vi "VisitLVType.vi"(8 "error in (no error)":errorcluster, 10 "LVType":refnum<class "LVType.lvclass">, 11 "NextGenXMLTypeGenerator in":refnum<class "NextGenXMLTypeGenerator.lvclass">) -> (0 "error out":errorcluster, 3 "NextGenXMLTypeGenerator out":refnum<class "NextGenXMLTypeGenerator.lvclass">)   [LabVIEW 2020, in "Web Service Description.lvlib" / "NextGenXMLTypeGenerator.lvclass"]
uses:
  <vilib>/AppBuilder/Engine/WebServiceDescription/NextGenXMLTypeGenerator/NextGenXMLTypeGenerator.lvclass
  <vilib>/AppBuilder/Engine/WebServiceDescription/LVDataTypes/LVType/LVType.lvclass
  <vilib>/AppBuilder/Engine/WebServiceDescription/XMLGen/ValuePair.ctl
  <vilib>/AppBuilder/Engine/WebServiceDescription/NextGenXMLTypeGenerator/NextGenXMLTypeGenerator.lvclass/NextGenXMLTypeGenerator.ctl
  <vilib>/AppBuilder/Engine/WebServiceDescription/XMLGen/XMLGen.lvlib
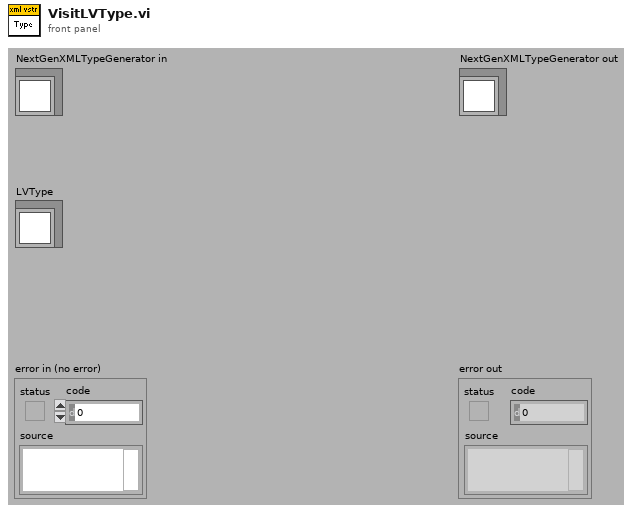
[diagram p1: front panel]
types:
  T1 = typedef "XMLGen.lvlib/ValuePair.ctl" = cluster{"Name":string, "Value":string}
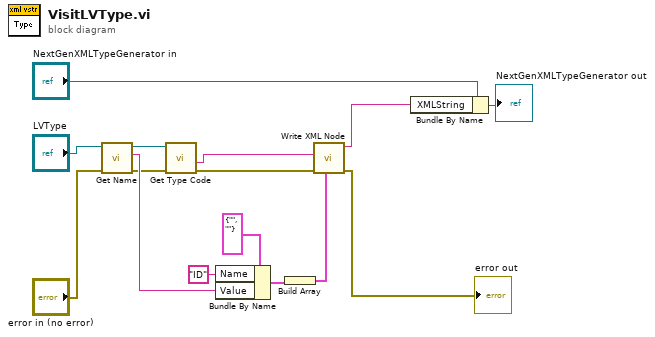
[diagram p0: block diagram]
diagram:
  n1 = call <vilib>:"Get Name.vi"("error in (no error)"="error in (no error)", "LVType.lvclass in"="LVType") -> ("error out"=w10:errorcluster, "Name"=w11:string, "LVType.lvclass out"=w9:refnum<class "LVType.lvclass">)  [unwired: 7 out]
  n2 = call <vilib>:"Get Type Code.vi"("error in (no error)"=w10, "LVType.lvclass in"=w9) -> ("error out"=w7:errorcluster, "TypeCodeString"=w8:string)  [unwired: 8 out]
  n3 = Bundle By Name(cluster=T1 {"Name"="", "Value"=""} ("Attribute"), "Name"="ID", "Value"=w11) -> (w6:T1)
  n4 = Build Array(w6) -> (w5:T1[])
  n5 = call <vilib>:"Write XML Node.vi"("attributes"=w5, "error in (no error)"=w7, "node"=w8) -> ("error out"=→"error out":errorcluster, "resulting string"=w3:string)  [unwired: 2 in, 5 out]
  n6 = Bundle By Name(cluster="NextGenXMLTypeGenerator in", "XMLString"=w3) -> (→"NextGenXMLTypeGenerator out":refnum<class "NextGenXMLTypeGenerator.lvclass">)
